vi "Close Scalar Refs.vi"(8 "error in (no error)":errorcluster, 11 "Cluster":T1 {"Data Type" format="%.0x"}) -> (0 "error out":errorcluster)   [LabVIEW 2018, in "FPGA Addon Engine.lvlib"]
uses:
  FPGA Addon Engine.lvlib
  <vilib>/rvi/interface/nirviCloseFPGA/nirviCloseFPGA.xnode
  <vilib>/FPGAPlugInAG/Dynamic/niLvFpga_Close_Dynamic.vi
  Types/Register Settings.ctl
  Addon Shared/Types/Scalar Type.ctl
  Addon Shared/FPGA Addon Shared.lvlib
  Addon Shared/Types/Data Type.ctl
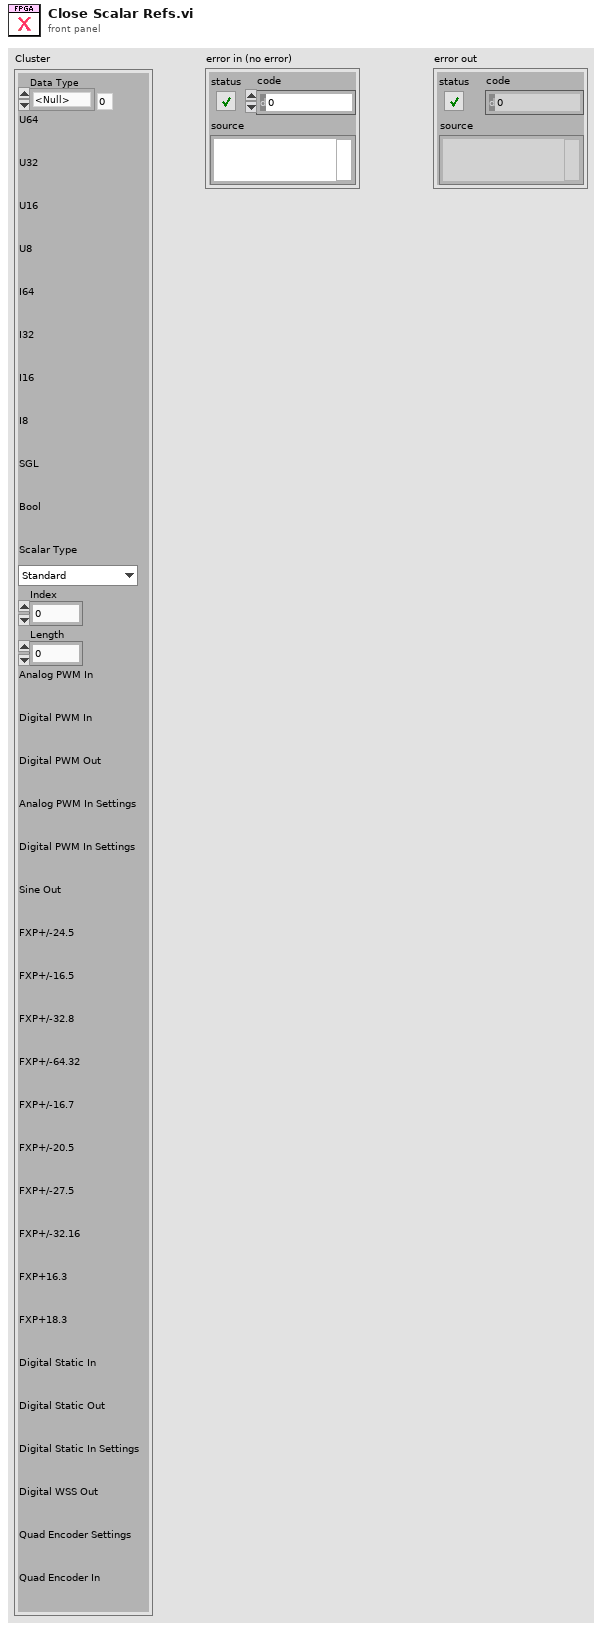
[diagram p1: front panel]
types:
  T1 = typedef "FPGA Addon Engine.lvlib/Register Settings.ctl" = cluster{"Data Type":T2, "U64":refnum<k20>, "U32":refnum<k20>, "U16":refnum<k20>, "U8":refnum<k20>, "I64":refnum<k20>, "I32":refnum<k20>, "I16":refnum<k20>, "I8":refnum<k20>, "SGL":refnum<k20>, "Bool":refnum<k20>, "Scalar Type":T3, "Index":i32, "Length":i32, "Analog PWM In":refnum<k20>, "Digital PWM In":refnum<k20>, "Digital PWM Out":refnum<k20>, "Analog PWM In Settings":refnum<k20>, "Digital PWM In Settings":refnum<k20>, "Sine Out":refnum<k20>, "FXP+/-24.5":refnum<k20>, "FXP+/-16.5":refnum<k20>, "FXP+/-32.8":refnum<k20>, "FXP+/-64.32":refnum<k20>, "FXP+/-16.7":refnum<k20>, "FXP+/-20.5":refnum<k20>, "FXP+/-27.5":refnum<k20>, "FXP+/-32.16":refnum<k20>, "FXP+16.3":refnum<k20>, "FXP+18.3":refnum<k20>, "Digital Static In":refnum<k20>, "Digital Static Out":refnum<k20>, "Digital Static In Settings":refnum<k20>, "Digital WSS Out":refnum<k20>, "Quad Encoder Settings":refnum<k20>, "Quad Encoder In":refnum<k20>}
  T2 = typedef "FPGA Addon Shared.lvlib/Data Type.ctl" = enum8{"<Null>", "I8", "I16", "I32", "I64", "U8", "U16", "U32", "U64", "SGL", "Boolean", "Analog PWM In Settings", "Analog PWM In", "Digital PWM In Settings", "Digital PWM In", "Digital PWM Out", "Sine Out", "FXP+/-24.5", "FXP+/-16.5", "FXP+/-32.8", "FXP+/-64.32", "FXP+/-16.7", "FXP+/-20.5", "FXP+/-27.5", "FXP+/-32.16", "FXP+16.3", "FXP+18.3", "Digital Static In", "Digital Static Out", "Digital Static In Settings", "Digital WSS Out", "Quad Encoder Settings", "Quad Encoder In", "Group"}
  T3 = typedef "FPGA Addon Shared.lvlib/Scalar Type.ctl" = enum16{"Standard", "Bitpacked"}
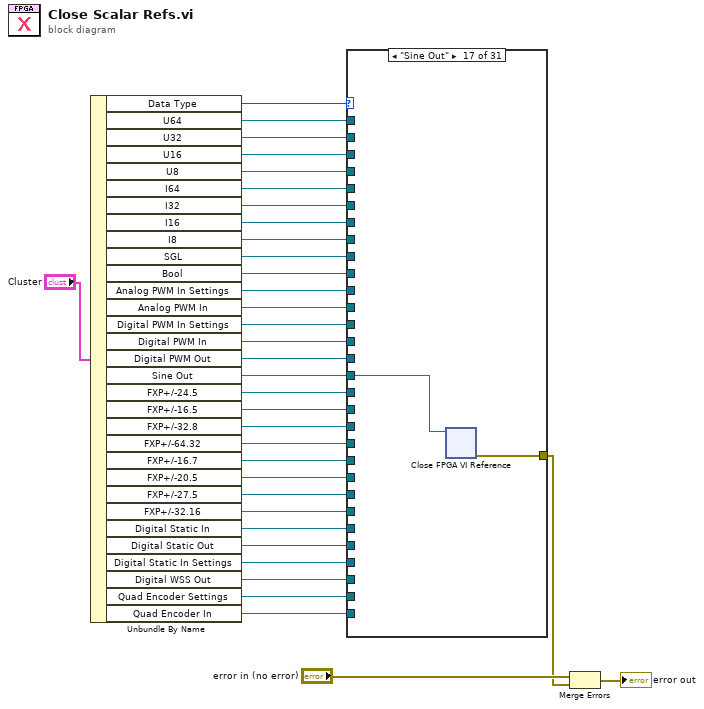
[diagram p0: block diagram]
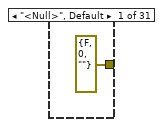
[diagram p2: hidden frame]
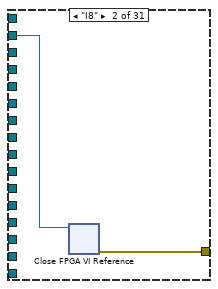
[diagram p3: hidden frame]
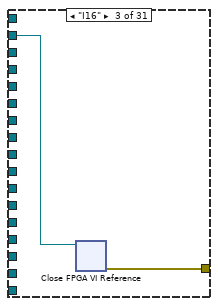
[diagram p4: hidden frame]
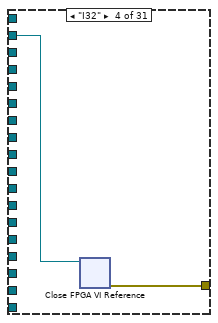
[diagram p5: hidden frame]
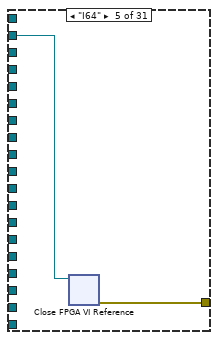
[diagram p6: hidden frame]
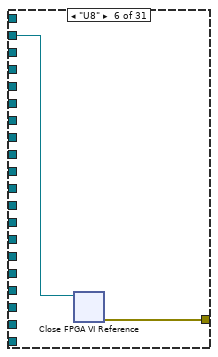
[diagram p7: hidden frame]
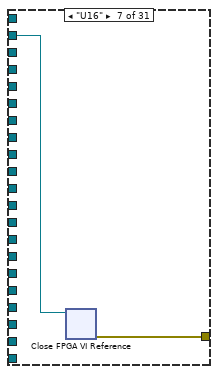
[diagram p8: hidden frame]
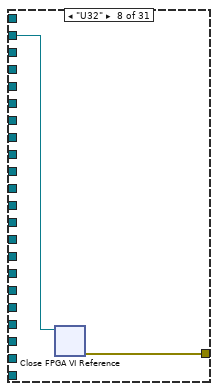
[diagram p9: hidden frame]
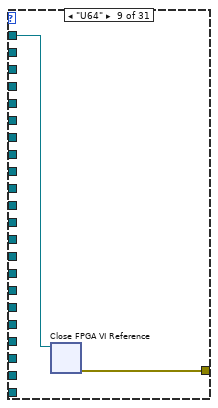
[diagram p10: hidden frame]
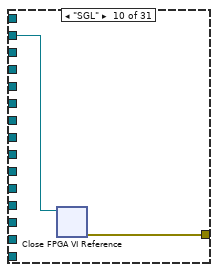
[diagram p11: hidden frame]
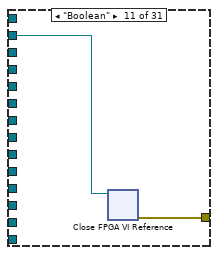
[diagram p12: hidden frame]
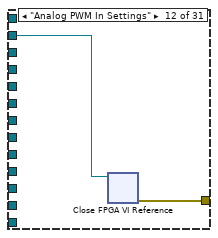
[diagram p13: hidden frame]
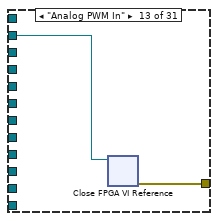
[diagram p14: hidden frame]
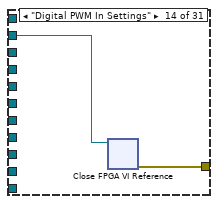
[diagram p15: hidden frame]
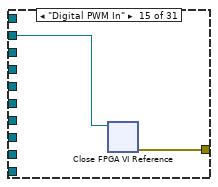
[diagram p16: hidden frame]
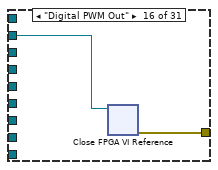
[diagram p17: hidden frame]
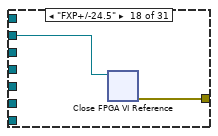
[diagram p18: hidden frame]
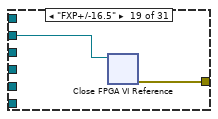
[diagram p19: hidden frame]
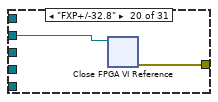
[diagram p20: hidden frame]
diagram:
  n1 = Unbundle By Name("Cluster") -> ("Data Type"=w35:T2, "U64"=w24:refnum<k20>, "U32"=w25:refnum<k20>, "U16"=w26:refnum<k20>, "U8"=w27:refnum<k20>, "I64"=w28:refnum<k20>, "I32"=w29:refnum<k20>, "I16"=w30:refnum<k20>, "I8"=w34:refnum<k20>, "SGL"=w32:refnum<k20>, "Bool"=w31:refnum<k20>, "Analog PWM In Settings"=w10:refnum<k20>, "Analog PWM In"=w11:refnum<k20>, "Digital PWM In Settings"=w12:refnum<k20>, "Digital PWM In"=w13:refnum<k20>, "Digital PWM Out"=w14:refnum<k20>, "Sine Out"=w15:refnum<k20>, "FXP+/-24.5"=w16:refnum<k20>, "FXP+/-16.5"=w17:refnum<k20>, "FXP+/-32.8"=w18:refnum<k20>, "FXP+/-64.32"=w19:refnum<k20>, "FXP+/-16.7"=w20:refnum<k20>, "FXP+/-20.5"=w9:refnum<k20>, "FXP+/-27.5"=w8:refnum<k20>, "FXP+/-32.16"=w7:refnum<k20>, "Digital Static In"=w6:refnum<k20>, "Digital Static Out"=w5:refnum<k20>, "Digital Static In Settings"=w4:refnum<k20>, "Digital WSS Out"=w3:refnum<k20>, "Quad Encoder Settings"=w2:refnum<k20>, "Quad Encoder In"=w1:refnum<k20>)
  n2 = case shown="\"Sine Out\"" w35 {
    tunnel: w34 -> [_ w37 _ _ _ _ _ _ _ _ _ _ _ _ _ _ _ _ _ _ _ _ _ _ _ _ _ _ _ _ _]
    tunnel: [errorcluster {"status"=FALSE, "code"=0, "source"=""} ("error out") w38 w40 w42 w44 w46 w48 w50 w52 w53 w56 w58 w60 w62 w64 w66 w68 w70 w72 w74 w76 w78 w80 w82 w84 w86 w88 w90 w92 w94 w96] -> w22
    tunnel: w32 -> [_ _ _ _ _ _ _ _ _ w54 _ _ _ _ _ _ _ _ _ _ _ _ _ _ _ _ _ _ _ _ _]
    tunnel: w31 -> [_ _ _ _ _ _ _ _ _ _ w55 _ _ _ _ _ _ _ _ _ _ _ _ _ _ _ _ _ _ _ _]
    tunnel: w30 -> [_ _ w39 _ _ _ _ _ _ _ _ _ _ _ _ _ _ _ _ _ _ _ _ _ _ _ _ _ _ _ _]
    tunnel: w29 -> [_ _ _ w41 _ _ _ _ _ _ _ _ _ _ _ _ _ _ _ _ _ _ _ _ _ _ _ _ _ _ _]
    tunnel: w28 -> [_ _ _ _ w43 _ _ _ _ _ _ _ _ _ _ _ _ _ _ _ _ _ _ _ _ _ _ _ _ _ _]
    tunnel: w27 -> [_ _ _ _ _ w45 _ _ _ _ _ _ _ _ _ _ _ _ _ _ _ _ _ _ _ _ _ _ _ _ _]
    tunnel: w26 -> [_ _ _ _ _ _ w47 _ _ _ _ _ _ _ _ _ _ _ _ _ _ _ _ _ _ _ _ _ _ _ _]
    tunnel: w25 -> [_ _ _ _ _ _ _ w49 _ _ _ _ _ _ _ _ _ _ _ _ _ _ _ _ _ _ _ _ _ _ _]
    tunnel: w24 -> [_ _ _ _ _ _ _ _ w51 _ _ _ _ _ _ _ _ _ _ _ _ _ _ _ _ _ _ _ _ _ _]
    tunnel: w20 -> [_ _ _ _ _ _ _ _ _ _ _ _ _ _ _ _ _ _ _ _ _ w77 _ _ _ _ _ _ _ _ _]
    tunnel: w19 -> [_ _ _ _ _ _ _ _ _ _ _ _ _ _ _ _ _ _ _ _ w75 _ _ _ _ _ _ _ _ _ _]
    tunnel: w18 -> [_ _ _ _ _ _ _ _ _ _ _ _ _ _ _ _ _ _ _ w73 _ _ _ _ _ _ _ _ _ _ _]
    tunnel: w17 -> [_ _ _ _ _ _ _ _ _ _ _ _ _ _ _ _ _ _ w71 _ _ _ _ _ _ _ _ _ _ _ _]
    tunnel: w16 -> [_ _ _ _ _ _ _ _ _ _ _ _ _ _ _ _ _ w69 _ _ _ _ _ _ _ _ _ _ _ _ _]
    tunnel: w15 -> [_ _ _ _ _ _ _ _ _ _ _ _ _ _ _ _ w67 _ _ _ _ _ _ _ _ _ _ _ _ _ _]
    tunnel: w14 -> [_ _ _ _ _ _ _ _ _ _ _ _ _ _ _ w65 _ _ _ _ _ _ _ _ _ _ _ _ _ _ _]
    tunnel: w13 -> [_ _ _ _ _ _ _ _ _ _ _ _ _ _ w63 _ _ _ _ _ _ _ _ _ _ _ _ _ _ _ _]
    tunnel: w12 -> [_ _ _ _ _ _ _ _ _ _ _ _ _ w61 _ _ _ _ _ _ _ _ _ _ _ _ _ _ _ _ _]
    tunnel: w11 -> [_ _ _ _ _ _ _ _ _ _ _ _ w59 _ _ _ _ _ _ _ _ _ _ _ _ _ _ _ _ _ _]
    tunnel: w10 -> [_ _ _ _ _ _ _ _ _ _ _ w57 _ _ _ _ _ _ _ _ _ _ _ _ _ _ _ _ _ _ _]
    tunnel: w9 -> [_ _ _ _ _ _ _ _ _ _ _ _ _ _ _ _ _ _ _ _ _ _ w79 _ _ _ _ _ _ _ _]
    tunnel: w8 -> [_ _ _ _ _ _ _ _ _ _ _ _ _ _ _ _ _ _ _ _ _ _ _ w81 _ _ _ _ _ _ _]
    tunnel: w7 -> [_ _ _ _ _ _ _ _ _ _ _ _ _ _ _ _ _ _ _ _ _ _ _ _ w83 _ _ _ _ _ _]
    tunnel: w6 -> [_ _ _ _ _ _ _ _ _ _ _ _ _ _ _ _ _ _ _ _ _ _ _ _ _ w85 _ _ _ _ _]
    tunnel: w5 -> [_ _ _ _ _ _ _ _ _ _ _ _ _ _ _ _ _ _ _ _ _ _ _ _ _ _ w87 _ _ _ _]
    tunnel: w4 -> [_ _ _ _ _ _ _ _ _ _ _ _ _ _ _ _ _ _ _ _ _ _ _ _ _ _ _ w89 _ _ _]
    tunnel: w3 -> [_ _ _ _ _ _ _ _ _ _ _ _ _ _ _ _ _ _ _ _ _ _ _ _ _ _ _ _ w91 _ _]
    tunnel: w2 -> [_ _ _ _ _ _ _ _ _ _ _ _ _ _ _ _ _ _ _ _ _ _ _ _ _ _ _ _ _ w93 _]
    tunnel: w1 -> [_ _ _ _ _ _ _ _ _ _ _ _ _ _ _ _ _ _ _ _ _ _ _ _ _ _ _ _ _ _ w95]
    frame "<Null>", Default {
    }
    frame "I8" {
      n3 = xnode "Close FPGA VI Reference"("FPGA VI Reference In"=w37) -> ("error out"=w38:errorcluster)  [unwired: 1 in]
    }
    frame "I16" {
      n4 = xnode "Close FPGA VI Reference"("FPGA VI Reference In"=w39) -> ("error out"=w40:errorcluster)  [unwired: 1 in]
    }
    frame "I32" {
      n5 = xnode "Close FPGA VI Reference"("FPGA VI Reference In"=w41) -> ("error out"=w42:errorcluster)  [unwired: 1 in]
    }
    frame "I64" {
      n6 = xnode "Close FPGA VI Reference"("FPGA VI Reference In"=w43) -> ("error out"=w44:errorcluster)  [unwired: 1 in]
    }
    frame "U8" {
      n7 = xnode "Close FPGA VI Reference"("FPGA VI Reference In"=w45) -> ("error out"=w46:errorcluster)  [unwired: 1 in]
    }
    frame "U16" {
      n8 = xnode "Close FPGA VI Reference"("FPGA VI Reference In"=w47) -> ("error out"=w48:errorcluster)  [unwired: 1 in]
    }
    frame "U32" {
      n9 = xnode "Close FPGA VI Reference"("FPGA VI Reference In"=w49) -> ("error out"=w50:errorcluster)  [unwired: 1 in]
    }
    frame "U64" {
      n10 = xnode "Close FPGA VI Reference"("FPGA VI Reference In"=w51) -> ("error out"=w52:errorcluster)  [unwired: 1 in]
    }
    frame "SGL" {
      n11 = xnode "Close FPGA VI Reference"("FPGA VI Reference In"=w54) -> ("error out"=w53:errorcluster)  [unwired: 1 in]
    }
    frame "Boolean" {
      n12 = xnode "Close FPGA VI Reference"("FPGA VI Reference In"=w55) -> ("error out"=w56:errorcluster)  [unwired: 1 in]
    }
    frame "Analog PWM In Settings" {
      n13 = xnode "Close FPGA VI Reference"("FPGA VI Reference In"=w57) -> ("error out"=w58:errorcluster)  [unwired: 1 in]
    }
    frame "Analog PWM In" {
      n14 = xnode "Close FPGA VI Reference"("FPGA VI Reference In"=w59) -> ("error out"=w60:errorcluster)  [unwired: 1 in]
    }
    frame "Digital PWM In Settings" {
      n15 = xnode "Close FPGA VI Reference"("FPGA VI Reference In"=w61) -> ("error out"=w62:errorcluster)  [unwired: 1 in]
    }
    frame "Digital PWM In" {
      n16 = xnode "Close FPGA VI Reference"("FPGA VI Reference In"=w63) -> ("error out"=w64:errorcluster)  [unwired: 1 in]
    }
    frame "Digital PWM Out" {
      n17 = xnode "Close FPGA VI Reference"("FPGA VI Reference In"=w65) -> ("error out"=w66:errorcluster)  [unwired: 1 in]
    }
    frame "Sine Out" {
      n18 = xnode "Close FPGA VI Reference"("FPGA VI Reference In"=w67) -> ("error out"=w68:errorcluster)  [unwired: 1 in]
    }
    frame "FXP+/-24.5" {
      n19 = xnode "Close FPGA VI Reference"("FPGA VI Reference In"=w69) -> ("error out"=w70:errorcluster)  [unwired: 1 in]
    }
    frame "FXP+/-16.5" {
      n20 = xnode "Close FPGA VI Reference"("FPGA VI Reference In"=w71) -> ("error out"=w72:errorcluster)  [unwired: 1 in]
    }
    frame "FXP+/-32.8" {
      n21 = xnode "Close FPGA VI Reference"("FPGA VI Reference In"=w73) -> ("error out"=w74:errorcluster)  [unwired: 1 in]
    }
    frame "FXP+/-64.32" {
      n22 = xnode "Close FPGA VI Reference"("FPGA VI Reference In"=w75) -> ("error out"=w76:errorcluster)  [unwired: 1 in]
    }
    frame "FXP+/-16.7" {
      n23 = xnode "Close FPGA VI Reference"("FPGA VI Reference In"=w77) -> ("error out"=w78:errorcluster)  [unwired: 1 in]
    }
    frame "FXP+/-20.5" {
      n24 = xnode "Close FPGA VI Reference"("FPGA VI Reference In"=w79) -> ("error out"=w80:errorcluster)  [unwired: 1 in]
    }
    frame "FXP+/-27.5" {
      n25 = xnode "Close FPGA VI Reference"("FPGA VI Reference In"=w81) -> ("error out"=w82:errorcluster)  [unwired: 1 in]
    }
    frame "FXP+/-32.16" {
      n26 = xnode "Close FPGA VI Reference"("FPGA VI Reference In"=w83) -> ("error out"=w84:errorcluster)  [unwired: 1 in]
    }
    frame "Digital Static In" {
      n27 = xnode "Close FPGA VI Reference"("FPGA VI Reference In"=w85) -> ("error out"=w86:errorcluster)  [unwired: 1 in]
    }
    frame "Digital Static Out" {
      n28 = xnode "Close FPGA VI Reference"("FPGA VI Reference In"=w87) -> ("error out"=w88:errorcluster)  [unwired: 1 in]
    }
    frame "Digital Static In Settings" {
      n29 = xnode "Close FPGA VI Reference"("FPGA VI Reference In"=w89) -> ("error out"=w90:errorcluster)  [unwired: 1 in]
    }
    frame "Digital WSS Out" {
      n30 = xnode "Close FPGA VI Reference"("FPGA VI Reference In"=w91) -> ("error out"=w92:errorcluster)  [unwired: 1 in]
    }
    frame "Quad Encoder Settings" {
      n31 = xnode "Close FPGA VI Reference"("FPGA VI Reference In"=w93) -> ("error out"=w94:errorcluster)  [unwired: 1 in]
    }
    frame "Quad Encoder In" {
      n32 = xnode "Close FPGA VI Reference"("FPGA VI Reference In"=w95) -> ("error out"=w96:errorcluster)  [unwired: 1 in]
    }
  }
  n33 = Merge Errors("error in (no error)", w22) -> (→"error out":errorcluster)
